vi "ELTA_Phase_Calibration.vi"() -> ()   [LabVIEW 2023, in "ELTA.lvlib"]
uses:
  ELTA.lvlib
  Anritsu Signal Analyzer Series/Anritsu Signal Analyzer Series.lvlib
panel:
  in  "Daul_Ch_Phase_Sweep":bool
  in  "SweepSwitch?":u16(ring) items=["Special", "Sweep"]
  in  "SweepMode":u16(ring) items=["Phase", "Gain"]
  in  "Method":u16(ring)=1 items=["dBm"=1, "mW"=2]
  in  "Polarity":u16(ring) items=["H", "V"]
  in  "VISA resource name":refnum<visa-resource-name>="TCPIP0::192.168.100.230::inst0::INSTR"
  in  "CenterFreq(GHz)":dbl=28.0
  in  "AvgTimes":i32=3
  in  "Single_Ch_Phase_Sweep":bool
  in  "TRXmode":u16(ring)=1 items=["Rx"=2, "Tx"=1]
  out "GainStep":i32=63
  out "PhaseStep":i32=63
  out "Channel":i32=63
  out "Total mW":dbl format="%.7f"
  out "Total dBm":dbl format="%.7f"
  out "Ref. mW":dbl format="%.7f"
  out "Ref. dBm":dbl format="%.7f"
  out "Main mW":dbl format="%.7f"
  out "Main dBm":dbl format="%.7f"
  out "Data":dbl[][](array[numeric])
  out "FileNAME_Single":string
  out "Spectrum Analyzer":dbl[](graph)
  out "CurrentData":dbl[](array[numeric])
  out "Duration":dbl
  out "TotalTime":dbl format="%.2f"
  out "StopTime":timestamp=timestamp(3663835912.033212 s since 1904-01-01)
  out "FileNAME_Dual":string
  out "StartTime":timestamp=timestamp(3663835741.875155 s since 1904-01-01)
  out "TX/RX":u16=1
  out "error out":errorcluster
  out "output cluster":T1={"address"="192.168.100.111", "remote port or service name"=5025, "timeout ms (60000)"=10000}
  out "Operating \nChannel(s)":bool[][](array[boolean])
  out "OK?":bool
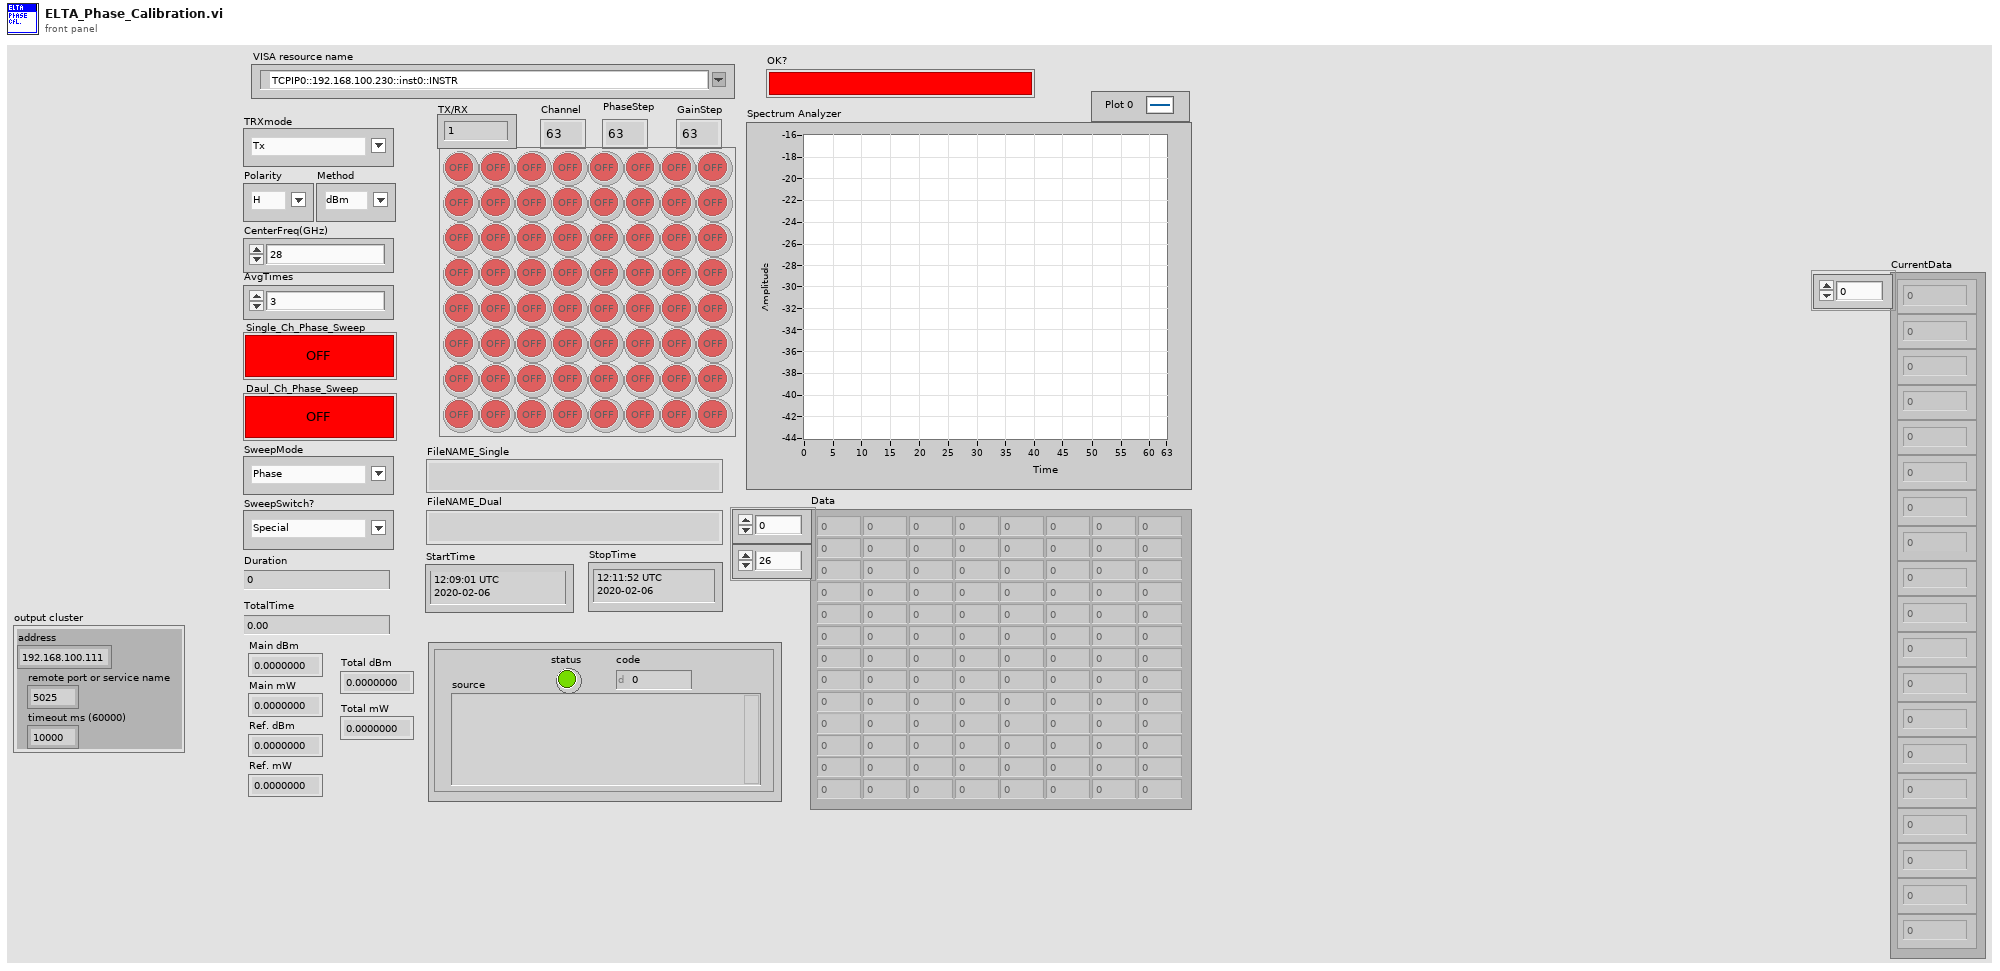
[diagram p1: front panel]
types:
  T1 = cluster{"address":string, "remote port or service name":u16, "timeout ms (60000)":i32}
  T2 = cluster{"Mode":u16, "Polarity":u16, "CH_ON/OFF":u16, "Channel":i32, "Gain":i32, "Phase":i32}
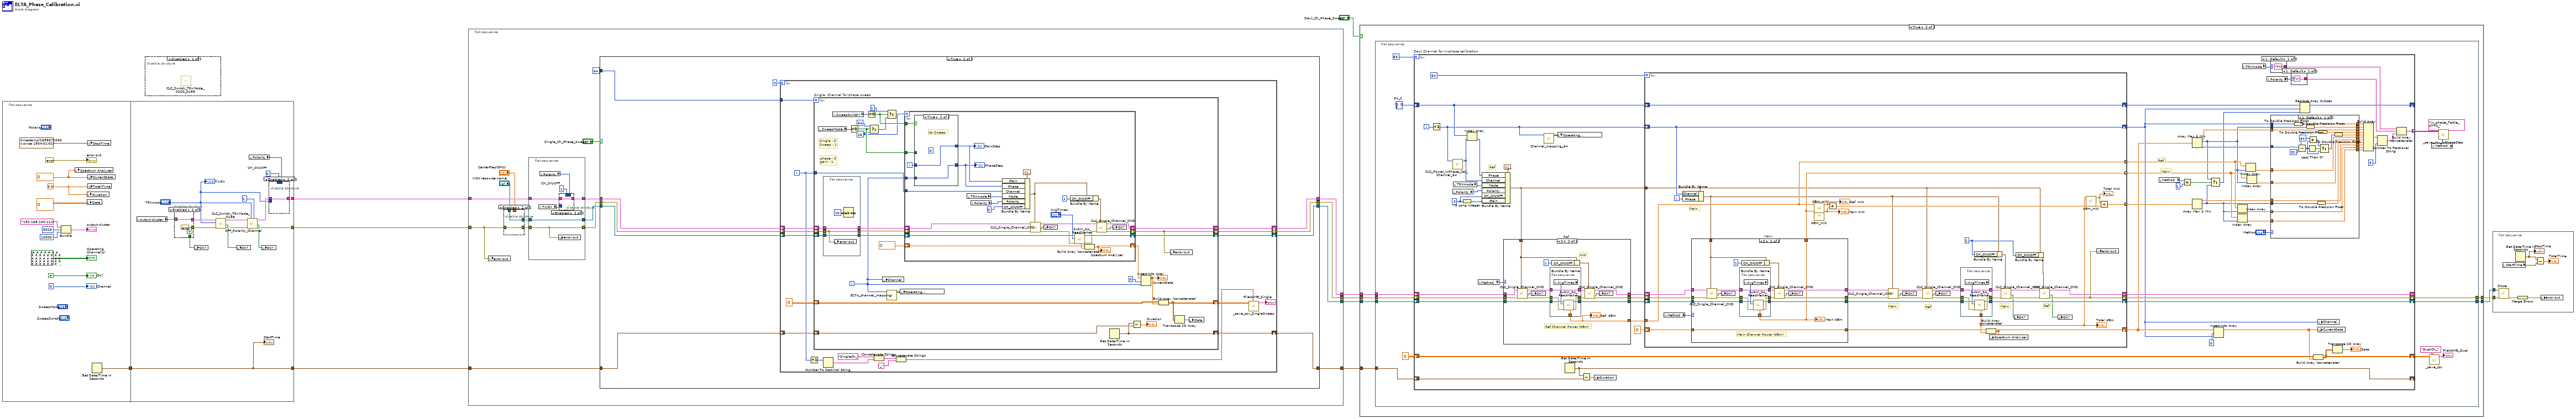
[diagram p0: block diagram]
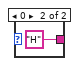
[diagram p4: hidden frame]
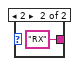
[diagram p5: hidden frame]
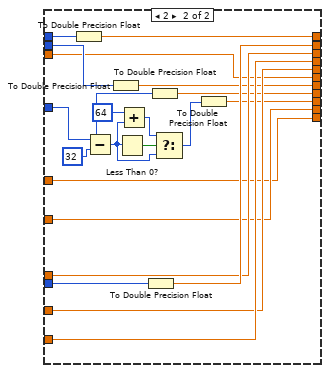
[diagram p6: hidden frame]
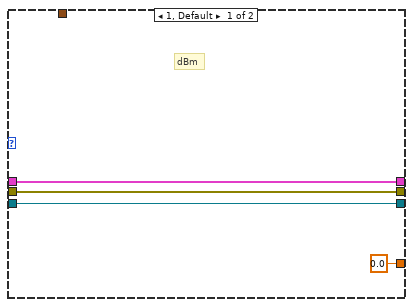
[diagram p7: hidden frame]
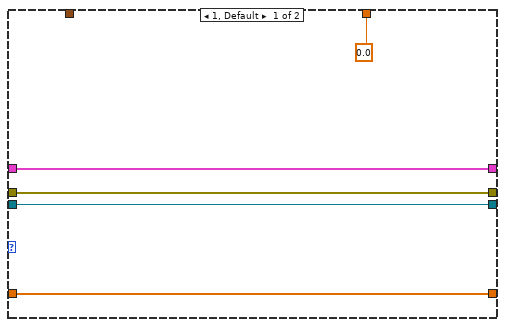
[diagram p8: hidden frame]
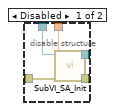
[diagram p9: hidden frame]
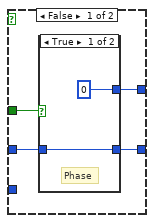
[diagram p11: hidden frame]
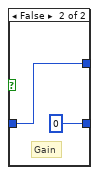
[diagram p12: hidden frame]
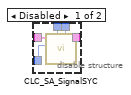
[diagram p13: hidden frame]
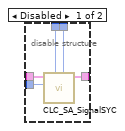
[diagram p14: hidden frame]
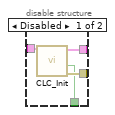
[diagram p15: hidden frame]
diagram:
  n1 = flat-sequence {
    tunnel: [w12] -> w11
    tunnel: w11 -> [w28]
    tunnel: [w31] -> w2
    tunnel: [w35] -> w3
    tunnel: [w28] -> w10
    frame #0 {
      w16 = dbl[] []
      w19 = 0.0 ("TotalTime")
      n2 = Bundle("address"="192.168.100.111", "remote port or service name"=u16 5025, "timeout ms (60000)"=10000) -> (→"output cluster":T1)  [unwired: 1 in]
      n3 = local write "Spectrum Analyzer"(w16) -> ()
      n4 = local write "Duration"(w19) -> ()
      n5 = local write "Data"(dbl[][] []) -> ()
      n6 = local write "StopTime"(timestamp(2658672000.001 s since 1904-01-01) ("StopTime")) -> ()
      n7 = local write "CurrentData"(w16) -> ()
      n8 = local write "TotalTime"(w19) -> ()
      n9 = Get Date/Time In Seconds() -> (seconds since 1Jan1904=w12:timestamp)
      "error out" <- errorcluster {"status"=FALSE, "code"=0, "source"=""} ("error out")
      "Operating \nChannel(s)" <- bool[][] [[FALSE, FALSE, FALSE, FALSE, FALSE, FALSE, FALSE, FALSE], [FALSE, FALSE, FALSE, FALSE, FALSE, FALSE, FALSE, FALSE], [FALSE, FALSE, FALSE, FALSE, FALSE, FALSE, FALSE, FALSE], [FALSE, FALSE, FALSE, FALSE, FALSE, FALSE, FALSE, FALSE], [FALSE, FALSE, FALSE, FALSE, FALSE, FALSE, FALSE, FALSE], [FALSE, FALSE, FALSE, FALSE, FALSE, FALSE, FALSE, FALSE], [FALSE, FALSE, FALSE, FALSE, FALSE, FALSE, FALSE, FALSE], [FALSE, FALSE, FALSE, FALSE, FALSE, FALSE, FALSE, FALSE]] ("Operating \nChannel(s)")
      "Channel" <- 0 ("Channel")
      "OK?" <- FALSE ("OK?")
    }
    frame #1 {
      w30 = u16 0  # CH_ON/OFF
      n10 = local read "output cluster"() -> (w40:T1)
      n11 = disable-structure shown="Enabled" {
        disable-tunnel: w40 -> [w50 w53]
        disable-tunnel: [w49 w53] -> w39
        disable-tunnel: [w48 errorcluster {"status"=FALSE, "code"=0, "source"=""} ("error in (no error)")] -> w37
        disable-tunnel: [w47 TRUE ("OK?")] -> w29
        frame Disabled {
          n12 = call "CLC_Init.vi"("TCPIPin"=w50) -> ("error out"=w48:errorcluster, "Status"=w47:bool, "TCPIPin 2"=w49:T1)  [unwired: 8 in]
        }
        frame Enabled {
        }
      }
      n13 = local write "OK?"(w29) -> ()
      n14 = call "CLC_Switch_TRxMode_0188.vi"("error in (no error)"=w37, "Text Ring"="TRXmode", "TCPIPin"=w39) -> ("error out"=w36:errorcluster, "OK?"=w38:bool, "TCPIPin 2"=w34:T1)  [unwired: 6 in]
      n15 = local write "OK?"(w38) -> ()
      n16 = call "OFF_Polarity_Channel.vi"("CH_ON:0/OFF:1"=u16 1, "Mode"="TRXmode", "error in"=w36, "TCPIPin"=w34) -> ("error out"=w35:errorcluster, "OK?"=w33:bool, "TCPIPout"=w32:T1)  [unwired: 5 in]
      n17 = local read "Polarity"() -> (w26:u16)
      n18 = local write "OK?"(w33) -> ()
      n19 = disable-structure shown="Enabled" {
        disable-tunnel: w32 -> [w45 w46]
        disable-tunnel: [w44 w46] -> w31
        disable-tunnel: w30 -> [w43 _]
        disable-tunnel: w26 -> [w42 _]
        disable-tunnel: "TRXmode" -> [w41 _]
        frame Disabled {
          n20 = call "CLC_SA_SignalSYC.vi"("Polarity"=w42, "CH_ON/OFF"=w43, "Mode"=w41, "TCPIPin"=w45) -> ("TCPIPout"=w44:T1)  [unwired: 7 in]
        }
        frame Enabled {
        }
      }
      "StartTime" <- w28
      "TX/RX" <- "TRXmode"
    }
  }
  n21 = disable-structure shown="Disabled" {
    frame Disabled {
      n22 = call "CLC_Switch_TRxMode_0200_0188.vi"() -> ()  [unwired: 9 in, 3 out]
    }
    frame Enabled {
    }
  }
  n23 = flat-sequence {
    tunnel: w10 -> [w67]
    tunnel: [w66] -> w9
    tunnel: [w65] -> w8
    tunnel: [w64] -> w7
    tunnel: [w63] -> w4
    tunnel: w3 -> [w61]
    tunnel: w2 -> [w58]
    frame #0 {
      n24 = local write "error out"(w61) -> ()
      n25 = disable-structure shown="Enabled" {
        disable-tunnel: "VISA resource name" -> [w74 w75]
        disable-tunnel: [w73 w76] -> w62
        disable-tunnel: w61 -> [w72 w76]
        disable-tunnel: "CenterFreq(GHz)" -> [w71 _]
        disable-tunnel: [w70 w75] -> w57
        frame Disabled {
          n26 = call "SubVI_SA_Init.vi"("error in (no error)"=w72, "CenterFreq(GHz) 2"=w71, "VISA resource name"=w74) -> ("error out 2"=w73:errorcluster, "VISA resource name out"=w70:refnum<visa-resource-name>)  [unwired: 6 in, 1 out]
        }
        frame Enabled {
        }
      }
      n27 = flat-sequence {
        tunnel: w62 -> [w189]
        tunnel: [w189] -> w59
        tunnel: w58 -> [w187]
        tunnel: w57 -> [w188]
        tunnel: [w188] -> w56
        tunnel: [w186] -> w55
        frame #0 {
          w185 = u16 1  # CH_ON/OFF
          n28 = local read "TX/RX"() -> (w183:u16)
          n29 = local read "Polarity"() -> (w184:u16)
          n30 = local write "error out"(w189) -> ()
          n31 = disable-structure shown="Enabled" {
            disable-tunnel: w187 -> [w194 w195]
            disable-tunnel: [w193 w195] -> w186
            disable-tunnel: w185 -> [w192 _]
            disable-tunnel: w184 -> [w191 _]
            disable-tunnel: w183 -> [w190 _]
            frame Disabled {
              n32 = call "CLC_SA_SignalSYC.vi"("Polarity"=w191, "CH_ON/OFF"=w192, "Mode"=w190, "TCPIPin"=w194) -> ("TCPIPout"=w193:T1)  [unwired: 7 in]
            }
            frame Enabled {
            }
          }
        }
      }
      n33 = case shown="True" "Single_Ch_Phase_Sweep" {
        tunnel: 64 -> [_ w90]
        tunnel: w67 -> [w77 w89]
        tunnel: [w78 w88] -> w66
        tunnel: [w79 w87] -> w65
        tunnel: [w80 w86] -> w64
        tunnel: [w77 w85] -> w63
        tunnel: w59 -> [w79 w84]
        tunnel: w56 -> [w78 w83]
        tunnel: w55 -> [w80 w82]
        frame False {
        }
        frame True {
          n34 = for {
            N: 4 -> [_]
            tunnel: w90 -> [w109]
            shift-right: [w104] -> w85
            shift-left: w89 -> [w108]
            shift-right: [w106] -> w87
            shift-left: w84 -> [w103]
            shift-right: [w107] -> w88
            shift-left: w83 -> [w102]
            shift-right: [w105] -> w86
            shift-left: w82 -> [w101]
            i -> [w97]
            n35 = Increment(x=w97) -> (x+1=w91:i32)
            n36 = for "Single  Channel for phase sweep" {
              N: w109 -> [_]
              shift-right: [w139] -> w105
              shift-left: w101 -> [w125]
              shift-right: [w134] -> w106
              shift-left: w103 -> [w127]
              shift-right: [w138] -> w107
              shift-left: w102 -> [w124]
              shift-right: [w132] -> w99
              shift-left: dbl[][] [] -> [w133]
              shift-right: [w136] -> w104
              shift-left: w108 -> [w135]
              tunnel: w97 -> [w111]
              i -> [w110]
              w112 = 16
              # "Single : 0\nSweep : 1"
              # "phase : 0\ngain : 1"
              n37 = local read "SweepMode"() -> (w119:u16)
              n38 = flat-sequence {
                tunnel: [w141] -> w123
                tunnel: w127 -> [w142]
                tunnel: [w142] -> w126
                tunnel: w125 -> [w141]
                tunnel: w124 -> [w140]
                tunnel: [w140] -> w122
                frame #0 {
                  n39 = local write "error out"(w142) -> ()
                  n40 = Wait (ms)(milliseconds to wait=u32 10) -> ()  [unwired: 1 out]
                }
              }
              n41 = local read "SweepSwitch?"() -> (w118:u16)
              n42 = Equal To 0?(x=w119) -> (x = 0?=w113:bool)
              n43 = Equal To 0?(x=w118) -> (x = 0?=w114:bool)
              n44 = Select(t=64, s=w113, f=w112) -> (s? t:f=w115:i32)
              n45 = local write "Channel"(w110) -> ()
              n46 = Select(t=1, s=w114, f=w115) -> ()  [unwired: 1 out]
              n47 = call "ELTA_channel_mapping.vi"("Ch_1_ref"=w110) -> ("Operating \nChannel(s)"=w120:bool[][])  [unwired: 10 in]
              n48 = local write "Operating \nChannel(s)"(w120) -> ()
              n49 = for {
                N: w112 -> [_]
                shift-right: [w154] -> w139
                shift-left: w123 -> [w164]
                shift-right: [w156] -> w134
                shift-left: w126 -> [w166]
                shift-right: [w171] -> w138
                shift-left: w122 -> [w172]
                shift-right: [w167] -> w131
                shift-left: dbl[] [] -> [w168]
                tunnel: w111 -> [w161]
                tunnel: w114 -> [w149]
                tunnel: w113 -> [w146]
                tunnel: w110 -> [w144]
                i -> [w145]
                n50 = case shown="True" w149 {
                  tunnel: [w173 w182] -> w148
                  tunnel: [w174 w181] -> w147
                  tunnel: w146 -> [w176 _]
                  tunnel: w145 -> [w175 w182]
                  tunnel: w144 -> [_ w181]
                  frame False {
                    n51 = case shown="True" w176 {
                      tunnel: w175 -> [w178 w179]
                      tunnel: [w178 0] -> w174
                      tunnel: [0 w179] -> w173
                      frame True {
                        # "Phase"
                      }
                      frame False {
                        # "Gain"
                      }
                    }
                  }
                  frame True {
                    (unwired) 0
                    # "No Sweep"
                  }
                }
                "PhaseStep" <- w147
                "GainStep" <- w148
                n52 = local read "TRXmode"() -> (w160:u16)
                n53 = local read "Polarity"() -> (w159:u16)
                n54 = Bundle By Name(cluster=T2 {"Mode"=1, "Polarity"=1, "CH_ON/OFF"=1, "Channel"=0, "Gain"=0, "Phase"=0} ("Channel params"), "Gain"=w148, "Phase"=w147, "Channel"=w161, "Mode"=w160, "Polarity"=w159, "CH_ON/OFF"=u16 0) -> (w153:T2)
                n55 = call "CLC_Single_Channel_CMD.vi"("Channel params"=w153, "error in"=w166, "TCPIPin"=w164) -> ("error out"=w165:errorcluster, "OK?"=w162:bool, "TCPIPout"=w155:T1)  [unwired: 6 in]
                n56 = local write "OK?"(w162) -> ()
                n57 = Bundle By Name(cluster=w153, "CH_ON/OFF"=u16 1) -> (w151:T2)
                n58 = call "SubVI_SA_ReadMarker.vi"("error in (no error)"=w165, "AvgTimes"="AvgTimes", "VISA resource name"=w172) -> ("error out"=w157:errorcluster, "VISA resource name out"=w171:refnum<visa-resource-name>, "Marker Power"=w169:dbl)  [unwired: 5 in, 1 out]
                n59 = Build Array (concatenate)(w168, w169) -> (w167:dbl[])
                "Spectrum Analyzer" <- w167
                n60 = call "CLC_Single_Channel_CMD.vi"("Channel params"=w151, "error in"=w157, "TCPIPin"=w155) -> ("error out"=w156:errorcluster, "OK?"=w150:bool, "TCPIPout"=w154:T1)  [unwired: 6 in]
                n61 = local write "OK?"(w150) -> ()
              }
              n62 = Get Date/Time In Seconds() -> (seconds since 1Jan1904=w136:timestamp)
              n63 = Subtract(x=w136, y=w135) -> (x-y=→"Duration":dbl)
              n64 = Insert Into Array(array=w131, index=0, new element=w110) -> (w129:dbl[])
              "CurrentData" <- w129
              n65 = Build Array (concatenate)(w133, w129) -> (w132:dbl[][])
              n66 = local write "error out"(w134) -> ()
              n67 = Transpose 2D Array(2D array=w132) -> (transposed array=w121:dbl[][])
              n68 = local write "Data"(w121) -> ()
            }
            n69 = Number To Decimal String(number=w91) -> (decimal integer string=w95:string)  [unwired: 1 in]
            n70 = Concatenate Strings("SingleCh_" ("delimiter (\\t)"), w95) -> (w94:string)
            n71 = Concatenate Strings(w94, "_") -> (w92:string)
            n72 = call "_save_csv_SingleSweep.vi"("delimiter (\\t)"=w92, "Data"=w99) -> ("FileName"=→"FileNAME_Single":string)  [unwired: 9 in]
          }
        }
      }
    }
  }
  n73 = case shown="True" "Daul_Ch_Phase_Sweep" {
    tunnel: w9 -> [w197 w203]
    tunnel: w8 -> [w196 w202]
    tunnel: w7 -> [_ w201]
    tunnel: [w197 w200] -> w6
    tunnel: [w196 w199] -> w5
    tunnel: w4 -> [_ w198]
    frame False {
    }
    frame True {
      n74 = flat-sequence {
        tunnel: w203 -> [w217]
        tunnel: w202 -> [w216]
        tunnel: w201 -> [w215]
        tunnel: [w214] -> w200
        tunnel: [w213] -> w199
        tunnel: w198 -> [w212]
        frame #0 {
          w210 = i32[] [0, 0, 0, 0, 0, 0, 0, 0, 0, 0, 0, 0, 0, 0, 0, 0, 0, 0, 0, 0, 0, 0, 0, 0, 0, 0, 0, 0, 0, 0, 0, 0, 0, 0, 0, 0, 0, 0, 0, 0, 0, 0, 0, 0, 0, 0, 0, 0, 0, 0, 0, 0, 0, 0, 0, 0, 0, 0, 0, 0, 0, 0, 0, 0]  # 64_0
          n75 = for "Daul Channel for in-phase calibration" {
            N: 63 -> [_]
            shift-right: [w291] -> _
            shift-left: w215 -> [w255]
            shift-right: [w288] -> w213
            shift-left: w216 -> [w259]
            shift-right: [w289] -> w214
            shift-left: w217 -> [w257]
            shift-right: [w283] -> w205
            shift-left: dbl[][] [] -> [w284]
            shift-right: [w287] -> _
            shift-left: w212 -> [w286]
            shift-right: [w277] -> _
            shift-left: w210 -> [w252]
            tunnel: [w221] -> w206 mode=indexing
            i -> [w220]
            w261 = u16 0 ("CH_ON/OFF")
            # "Main"
            # "Ref."
            # "Ref"
            n76 = Increment(x=w220) -> (x+1=w219:i32)
            n77 = call "CLC_Power_InPhase_Cal_Channel_64.vi"("Channel IN"=w219) -> ("Ref_Channel"=w248:i32)  [unwired: 8 in, 2 out]
            n78 = local read "Polarity"() -> (w262:u16)
            n79 = local read "TRXmode"() -> (w263:u16)
            n80 = To Long Integer(number=w261) -> (32bit integer=w260:i32)
            n81 = Index Array(array=w252, index=w248) -> (element=w251:i32)
            n82 = local read "Method"() -> (w249:u16)
            n83 = Bundle By Name(cluster=T2 {"Mode"=1, "Polarity"=1, "CH_ON/OFF"=1, "Channel"=0, "Gain"=0, "Phase"=0} ("Channel params"), "Phase"=w251, "Channel"=w248, "Mode"=w263, "Polarity"=w262, "CH_ON/OFF"=w261, "Gain"=w260) -> (w250:T2)
            n84 = case "Ref" shown="2" w249 {
              tunnel: w259 -> [w340 w349]
              tunnel: [w340 w348] -> w258
              tunnel: w257 -> [w339 w347]
              tunnel: [w339 w346] -> w256
              tunnel: w255 -> [w341 w345]
              tunnel: [w341 w344] -> w254
              tunnel: [0.0 ("Marker Response") w343] -> w253
              tunnel: w250 -> [_ w342]
              frame 1, Default {
                # "dBm"
              }
              frame 2 {
                # "mW"
                # "Ref Channel Power (dBm)"
                n85 = call "CLC_Single_Channel_CMD.vi"("Channel params"=w342, "error in"=w349, "TCPIPin"=w345) -> ("error out"=w356:errorcluster, "OK?"=w357:bool, "TCPIPout"=w355:T1)  [unwired: 6 in]
                n86 = local write "OK?"(w357) -> ()
                n87 = flat-sequence {
                  tunnel: [w364] -> w346
                  tunnel: [w362] -> w343
                  tunnel: w347 -> [w361]
                  tunnel: w356 -> [w360]
                  tunnel: [w359] -> w351
                  tunnel: w355 -> [w359]
                  tunnel: [w358] -> w352
                  frame #0 {
                    n88 = local read "AvgTimes"() -> (w363:i32)
                    n89 = call "SubVI_SA_ReadMarker.vi"("error in (no error)"=w360, "AvgTimes"=w363, "VISA resource name"=w361) -> ("error out"=w358:errorcluster, "VISA resource name out"=w364:refnum<visa-resource-name>, "Marker Power"=w362:dbl)  [unwired: 5 in, 1 out]
                  }
                }
                n90 = Bundle By Name(cluster=w342, "CH_ON/OFF"=u16 1) -> (w353:T2)
                n91 = call "CLC_Single_Channel_CMD.vi"("Channel params"=w353, "error in"=w352, "TCPIPin"=w351) -> ("error out"=w348:errorcluster, "OK?"=w354:bool, "TCPIPout"=w344:T1)  [unwired: 6 in]
                n92 = local write "OK?"(w354) -> ()
                "Ref. dBm" <- w343
              }
            }
            n93 = call "Channel_mapping_64.vi"("Channel IN"=w219) -> ("Operating \nChannel(s)"=w265:bool[][])  [unwired: 10 in]
            n94 = local write "Operating \nChannel(s)"(w265) -> ()
            n95 = Get Date/Time In Seconds() -> (seconds since 1Jan1904=w287:timestamp)
            n96 = Subtract(x=w287, y=w286) -> (x-y=w285:dbl)
            n97 = local write "Duration"(w285) -> ()
            n98 = for {
              N: 64 -> [_]
              shift-right: [w390] -> w291
              shift-left: w254 -> [w373]
              shift-right: [w394] -> w288
              shift-left: w258 -> [w386]
              shift-right: [w405] -> w289
              shift-left: w256 -> [w385]
              shift-right: [w388] -> w278
              shift-left: dbl[] [] -> [w375]
              shift-right: [w399] -> w276
              shift-left: w252 -> [w399]
              shift-right: [w368] -> w275
              shift-left: w219 -> [w368]
              tunnel: [w372] -> w268 mode=indexing
              tunnel: [w379] -> w267 mode=indexing
              tunnel: [w380] -> w274 mode=indexing
              tunnel: w250 -> [w366]
              tunnel: w253 -> [w372]
              i -> [w369]
              w365 = u16 1 ("CH_ON/OFF")
              # "Main"
              # "Ref"
              # "Main"
              # "Ref"
              # "Main"
              n99 = local read "Method"() -> (w376:u16)
              n100 = Bundle By Name(cluster=w366, "Channel"=w368, "Phase"=w369) -> (w367:T2)
              n101 = case "Main" shown="2" w376 {
                tunnel: w386 -> [w408 w414]
                tunnel: w373 -> [w409 w415]
                tunnel: w385 -> [w407 w413]
                tunnel: [w409 w419] -> w384
                tunnel: [w408 w418] -> w383
                tunnel: [w407 w417] -> w382
                tunnel: w367 -> [_ w416]
                tunnel: [0.0 ("Marker Response") w411] -> w379
                tunnel: w375 -> [w406 w412]
                tunnel: [w406 w412] -> w374
                frame 1, Default {
                }
                frame 2 {
                  # "Main Channel Power (dBm)"
                  n102 = call "CLC_Single_Channel_CMD.vi"("Channel params"=w416, "error in"=w414, "TCPIPin"=w415) -> ("error out"=w421:errorcluster, "OK?"=w420:bool, "TCPIPout"=w422:T1)  [unwired: 6 in]
                  n103 = local write "OK?"(w420) -> ()
                  n104 = flat-sequence {
                    tunnel: [w434] -> w417
                    tunnel: [w432] -> w411
                    tunnel: w413 -> [w431]
                    tunnel: w421 -> [w430]
                    tunnel: [w429] -> w427
                    tunnel: w422 -> [w429]
                    tunnel: [w428] -> w426
                    frame #0 {
                      n105 = local read "AvgTimes"() -> (w433:i32)
                      n106 = call "SubVI_SA_ReadMarker.vi"("error in (no error)"=w430, "AvgTimes"=w433, "VISA resource name"=w431) -> ("error out"=w428:errorcluster, "VISA resource name out"=w434:refnum<visa-resource-name>, "Marker Power"=w432:dbl)  [unwired: 5 in, 1 out]
                    }
                  }
                  n107 = Bundle By Name(cluster=w416, "CH_ON/OFF"=u16 1) -> (w425:T2)
                  n108 = call "CLC_Single_Channel_CMD.vi"("Channel params"=w425, "error in"=w426, "TCPIPin"=w427) -> ("error out"=w418:errorcluster, "OK?"=w423:bool, "TCPIPout"=w419:T1)  [unwired: 6 in]
                  n109 = local write "OK?"(w423) -> ()
                  "Main dBm" <- w411
                }
              }
              n110 = call "dBm_mW.vi"("dBm"=w372) -> ("mW"=w371:dbl)  [unwired: 10 in]
              "Ref. mW" <- w371
              n111 = call "dBm_mW.vi"("dBm"=w379) -> ("mW"=w370:dbl)  [unwired: 10 in]
              "Main mW" <- w370
              n112 = Add(x=w371, y=w370) -> (x+y=w381:dbl)
              n113 = call "CLC_Single_Channel_CMD.vi"("Channel params"=w367, "error in"=w383, "TCPIPin"=w384) -> ("error out"=w403:errorcluster, "OK?"=w402:bool, "TCPIPout"=w404:T1)  [unwired: 6 in]
              n114 = local write "OK?"(w402) -> ()
              n115 = call "CLC_Single_Channel_CMD.vi"("Channel params"=w366, "error in"=w403, "TCPIPin"=w404) -> ("error out"=w400:errorcluster, "OK?"=w401:bool, "TCPIPout"=w398:T1)  [unwired: 6 in]
              n116 = local write "OK?"(w401) -> ()
              n117 = flat-sequence {
                tunnel: [w441] -> w405
                tunnel: [w439] -> w378
                tunnel: w382 -> [w438]
                tunnel: w400 -> [w437]
                tunnel: [w436] -> w397
                tunnel: w398 -> [w436]
                tunnel: [w435] -> w387
                frame #0 {
                  n118 = local read "AvgTimes"() -> (w440:i32)
                  n119 = call "SubVI_SA_ReadMarker.vi"("error in (no error)"=w437, "AvgTimes"=w440, "VISA resource name"=w438) -> ("error out"=w435:errorcluster, "VISA resource name out"=w441:refnum<visa-resource-name>, "Marker Power"=w439:dbl)  [unwired: 5 in, 1 out]
                }
              }
              n120 = Bundle By Name(cluster=w367, "CH_ON/OFF"=w365) -> (w389:T2)
              n121 = Build Array (concatenate)(w374, w378) -> (w388:dbl[])
              n122 = local write "Spectrum Analyzer"(w388) -> ()
              n123 = call "CLC_Single_Channel_CMD.vi"("Channel params"=w389, "error in"=w387, "TCPIPin"=w397) -> ("error out"=w395:errorcluster, "OK?"=w396:bool, "TCPIPout"=w393:T1)  [unwired: 6 in]
              n124 = local write "OK?"(w396) -> ()
              n125 = Bundle By Name(cluster=w366, "CH_ON/OFF"=w365) -> (w392:T2)
              n126 = call "CLC_Single_Channel_CMD.vi"("Channel params"=w392, "error in"=w395, "TCPIPin"=w393) -> ("error out"=w394:errorcluster, "OK?"=w391:bool, "TCPIPout"=w390:T1)  [unwired: 6 in]
              n127 = local write "OK?"(w391) -> ()
              n128 = call "dBm_mW.vi"("dBm"=w378) -> ("mW"=w377:dbl)  [unwired: 10 in]
              "Total mW" <- w377
              n129 = local write "error out"(w394) -> ()
              n130 = Divide(x=w377, y=w381) -> (x/y=w380:dbl)
              "Total dBm" <- w378
            }
            n131 = local read "Method"() -> (w235:u16)
            n132 = Equal?(x=w235, y=u16 1) -> (x = y?=w233:bool)
            n133 = Array Max & Min(array=w278) -> (max value=w245:dbl, max index (indices)=w232:i32, min index (indices)=w266:i32)  [unwired: 1 out]
            n134 = Array Max & Min(array=w274) -> (max value=w239:dbl, max index (indices)=w231:i32)  [unwired: 2 out]
            n135 = Select(t=w232, s=w233, f=w231) -> (s? t:f=w230:i32)
            n136 = Insert Into Array(array=w278, index=0, new element=w275) -> (w279:dbl[])
            n137 = Index Array(array=w268, index=w231) -> (element=w238:dbl)
            n138 = Index Array(array=w267, index=w231) -> (element=w237:dbl)
            n139 = local read "TRXmode"() -> (w226:u16)
            n140 = Index Array(array=w268, index=w232) -> (element=w243:dbl)
            n141 = Index Array(array=w267, index=w232) -> (element=w242:dbl)
            n142 = local read "Polarity"() -> (w225:u16)
            n143 = case shown="1, Default" w226 {
              tunnel: ["TX" "RX"] -> w222
              frame 1, Default {
              }
              frame 2 {
              }
            }
            n144 = case shown="1, Default" "Method" {
              tunnel: w275 -> [w310 w331]
              tunnel: [w296 w325] -> w273
              tunnel: [w309 w324] -> w272
              tunnel: [w308 w323] -> w271
              tunnel: [w307 w327] -> w270
              tunnel: [w306 w320] -> w269
              tunnel: w266 -> [w305 w330]
              tunnel: w231 -> [w304 w329]
              tunnel: w232 -> [w303 w328]
              tunnel: w245 -> [w296 w322]
              tunnel: [w297 w326] -> w246
              tunnel: [w302 w322] -> w244
              tunnel: w243 -> [w302 w317]
              tunnel: w242 -> [w301 w318]
              tunnel: [w301 w321] -> w241
              tunnel: [w300 w319] -> w240
              tunnel: w239 -> [w300 w325]
              tunnel: w238 -> [w299 w323]
              tunnel: w237 -> [w298 w324]
              tunnel: [w298 w317] -> w236
              tunnel: [w299 w318] -> w229
              frame 1, Default {
                n145 = To Double Precision Float(number=w310) -> (double precision float=w307:dbl)
                n146 = Subtract(x=w305, y=32) -> (x-y=w312:i32)
                n147 = To Double Precision Float(number=w303) -> (double precision float=w297:dbl)
                n148 = Less Than 0?(x=w312) -> (x < 0?=w315:bool)
                n149 = Add(x=64, y=w312) -> (x+y=w313:i32)
                n150 = To Double Precision Float(number=w304) -> (double precision float=w306:dbl)
                n151 = To Double Precision Float(number=w305) -> (double precision float=w309:dbl)
                n152 = Select(t=w313, s=w315, f=w312) -> (s? t:f=w311:i32)
                n153 = To Double Precision Float(number=w311) -> (double precision float=w308:dbl)
              }
              frame 2 {
                n154 = To Double Precision Float(number=w331) -> (double precision float=w327:dbl)
                n155 = Subtract(x=w330, y=32) -> (x-y=w333:i32)
                n156 = To Double Precision Float(number=w328) -> (double precision float=w321:dbl)
                n157 = Less Than 0?(x=w333) -> (x < 0?=w336:bool)
                n158 = Add(x=64, y=w333) -> (x+y=w334:i32)
                n159 = To Double Precision Float(number=w329) -> (double precision float=w326:dbl)
                n160 = To Double Precision Float(number=w330) -> (double precision float=w320:dbl)
                n161 = Select(t=w334, s=w336, f=w333) -> (s? t:f=w332:i32)
                n162 = To Double Precision Float(number=w332) -> (double precision float=w319:dbl)
              }
            }
            n163 = case shown="1, Default" w225 {
              tunnel: ["V" "H"] -> w223
              frame 1, Default {
              }
              frame 0 {
              }
            }
            n164 = Replace Array Subset(array=w276, new element=w230, index=w275) -> (w277:i32[])
            n165 = Build Array (concatenate)(w284, w279) -> (w283:dbl[][])
            n166 = local write "CurrentData"(w279) -> ()
            n167 = local write "Channel"(w275) -> ()
            n168 = Transpose 2D Array(2D array=w283) -> (transposed array=→"Data":dbl[][])
            n169 = Build Array(w270, w246, w273, w272, w271, w244, w241, w269, w240, w229, w236) -> (w227:dbl[])
            n170 = Number To Fractional String(number=w227, precision (6)=i16 3) -> (F-format string=w224:string[])  [unwired: 2 in]
            n171 = Build Array (concatenate)(w222, w223, w224) -> (w221:string[])
          }
          n172 = call "_save_csv.vi"("delimiter (\\t)"="DualCh_" ("delimiter (\\t)"), "Data"=w205) -> ("FileName"=→"FileNAME_Dual":string)  [unwired: 9 in]
          n173 = local read "Method"() -> (w204:u16)
          n174 = call "_save_csv_InPhaseStep.vi"("Method"=w204, "delimiter (\\t)"="In_phase_Table_CTTC_" ("delimiter (\\t)"), "dataInput"=w206) -> ()  [unwired: 8 in, 1 out]
        }
      }
    }
  }
  n175 = flat-sequence {
    tunnel: w6 -> [w447]
    tunnel: w5 -> [w446]
    frame #0 {
      n176 = call "Close.vi"("error in (no error)"=w446, "VISA resource name"=w447) -> ("error out"=w448:errorcluster)  [unwired: 9 in]
      n177 = local read "StartTime"() -> (w442:timestamp)
      n178 = Get Date/Time In Seconds() -> (seconds since 1Jan1904=w443:timestamp)
      "StopTime" <- w443
      n179 = Merge Errors(w448) -> (w445:errorcluster)
      n180 = Subtract(x=w443, y=w442) -> (x-y=→"TotalTime":dbl)
      n181 = local write "error out"(w445) -> ()
    }
  }
